vi "Main-top_feature.vi"() -> ()   [LabVIEW 2015]
uses:
  <vilib>/Utility/file.llb/Read Delimited Spreadsheet (string).vi
  <vilib>/Utility/file.llb/Write Delimited Spreadsheet (string).vi
  <vilib>/vision/NI_Vision_Development_Module.lvlib
  greenDet.dll
panel:
  out "element":string
  in  "Date Path":path=path "K:/Sort/TV/path - 副本.txt"
  in  "Image Main Path":path=path "K:/Sort/TV"
  in  "Save Base Path":path=path "K:/Sort/TV/1-Result"
  out "交集图":T1(plugin-control)
  out "交集像素个数":dbl
  in  "Pixel Measurements 2":T2[](array[typedef])=[35] items=["Center of Mass X", "Center of Mass Y", "First Pixel X", "First Pixel Y", "Bounding Rect Left", "Bounding Rect Top", "Bounding Rect Right", "Bounding Rect Bottom", "Max Feret Diameter Start X", "Max Feret Diameter Start Y", "Max Feret Diameter End X", "Max Feret Diameter End Y", "Max Horiz. Segment Length Left", "Max Horiz. Segment Length Right", "Max Horiz. Segment Length Row", "-", "Bounding Rect Width", "Bounding Rect Height", "Bounding Rect Diagonal", "Perimeter", "Convex Hull Perimeter", "Holes' Perimeter", "Max Feret Diameter", "Equivalent Ellipse Major Axis", "Equivalent Ellipse Minor Axis", "Equivalent Ellipse Minor Axis (Feret)", "Equivalent Rect Long Side", "Equivalent Rect Short Side", "Equivalent Rect Diagonal", "Equivalent Rect Short Side (Feret)", "Average Horiz. Segment Length", "Average Vert. Segment Length", "Hydraulic Radius", "Waddel Disk Diameter", "-", "Area", "Holes' Area", "Particle & Holes' Area", "Convex Hull Area", "Image Area", "-", "Number of Holes", "Number of Horiz. Segments", "Number of Vert. Segments", "-", "Orientation", "Max Feret Diameter Orientation", "-", "% Area/Image Area", "% Area/(Particle & Holes' Area)", "Ratio of Equivalent Ellipse Axes", "Ratio of Equivalent Rect Sides", "-", "Elongation Factor", "Compactness Factor", "Heywood Circularity Factor", "Type Factor", "-", "Sum X", "Sum Y", "Sum XX", "Sum XY", "Sum YY", "Sum XXX", "Sum XXY", "Sum XYY", "Sum YYY", "-", "Moment of Inertia XX", "Moment of Inertia XY", "Moment of Inertia YY", "Moment of Inertia XXX", "Moment of Inertia XXY", "Moment of Inertia XYY", "Moment of Inertia YYY", "Norm. Moment of Inertia XX", "Norm. Moment of Inertia XY", "Norm. Moment of Inertia YY", "Norm. Moment of Inertia XXX", "Norm. Moment of Inertia XXY", "Norm. Moment of Inertia XYY", "Norm. Moment of Inertia YYY", "Hu Moment 1", "Hu Moment 2", "Hu Moment 3", "Hu Moment 4", "Hu Moment 5", "Hu Moment 6", "Hu Moment 7"]
  in  "Pixel Measurements":T2[](array[typedef])=[35] items=["Center of Mass X", "Center of Mass Y", "First Pixel X", "First Pixel Y", "Bounding Rect Left", "Bounding Rect Top", "Bounding Rect Right", "Bounding Rect Bottom", "Max Feret Diameter Start X", "Max Feret Diameter Start Y", "Max Feret Diameter End X", "Max Feret Diameter End Y", "Max Horiz. Segment Length Left", "Max Horiz. Segment Length Right", "Max Horiz. Segment Length Row", "-", "Bounding Rect Width", "Bounding Rect Height", "Bounding Rect Diagonal", "Perimeter", "Convex Hull Perimeter", "Holes' Perimeter", "Max Feret Diameter", "Equivalent Ellipse Major Axis", "Equivalent Ellipse Minor Axis", "Equivalent Ellipse Minor Axis (Feret)", "Equivalent Rect Long Side", "Equivalent Rect Short Side", "Equivalent Rect Diagonal", "Equivalent Rect Short Side (Feret)", "Average Horiz. Segment Length", "Average Vert. Segment Length", "Hydraulic Radius", "Waddel Disk Diameter", "-", "Area", "Holes' Area", "Particle & Holes' Area", "Convex Hull Area", "Image Area", "-", "Number of Holes", "Number of Horiz. Segments", "Number of Vert. Segments", "-", "Orientation", "Max Feret Diameter Orientation", "-", "% Area/Image Area", "% Area/(Particle & Holes' Area)", "Ratio of Equivalent Ellipse Axes", "Ratio of Equivalent Rect Sides", "-", "Elongation Factor", "Compactness Factor", "Heywood Circularity Factor", "Type Factor", "-", "Sum X", "Sum Y", "Sum XX", "Sum XY", "Sum YY", "Sum XXX", "Sum XXY", "Sum XYY", "Sum YYY", "-", "Moment of Inertia XX", "Moment of Inertia XY", "Moment of Inertia YY", "Moment of Inertia XXX", "Moment of Inertia XXY", "Moment of Inertia XYY", "Moment of Inertia YYY", "Norm. Moment of Inertia XX", "Norm. Moment of Inertia XY", "Norm. Moment of Inertia YY", "Norm. Moment of Inertia XXX", "Norm. Moment of Inertia XXY", "Norm. Moment of Inertia XYY", "Norm. Moment of Inertia YYY", "Hu Moment 1", "Hu Moment 2", "Hu Moment 3", "Hu Moment 4", "Hu Moment 5", "Hu Moment 6", "Hu Moment 7"]
  out "黄色分量（油菜花）二值图":T1(plugin-control)
  out "黄色分量（油菜花）":T1(plugin-control)
  out "Original Image":T1(plugin-control)
  out "Current Path":path
  out "Current Number":string
  in  "ROI_whole":T3={"Top"=550, "im_height"=1000, "L_left"=650, "im_width"=1050}
  in  "Crop image ?":bool
  out "HistStat_whole":dbl[](array[numeric])
  out "AC (Area Convexity)":dbl
  out "P":dbl
  out "TPA (Total projective area)":dbl
  out "SFD":sgl
  out "BW (minimum circumscribed box width)":dbl
  out "BH":dbl
  out "R (Rectangularity)":dbl
  out "IFD":sgl
  out "Hull area":dbl
  out "HWR":dbl
  out "greenDet":dbl
  out "Crop Image":T1(plugin-control)
  out "Binary Image":T1(plugin-control)
  in  "EG threshold":sgl=0.2
  in  "ER threshold":sgl=0.5
  out "移除小区域后图像":T1(plugin-control)
  out "叶片分割后图像":T1(plugin-control)
  out "GPA (Green projective area)":dbl
  out "YPA (Yellow projective area)":dbl
  out "Image Path":path
  # "Digital evaluation software for oilseed rape phenotype-related traits (top-view) v1.0"
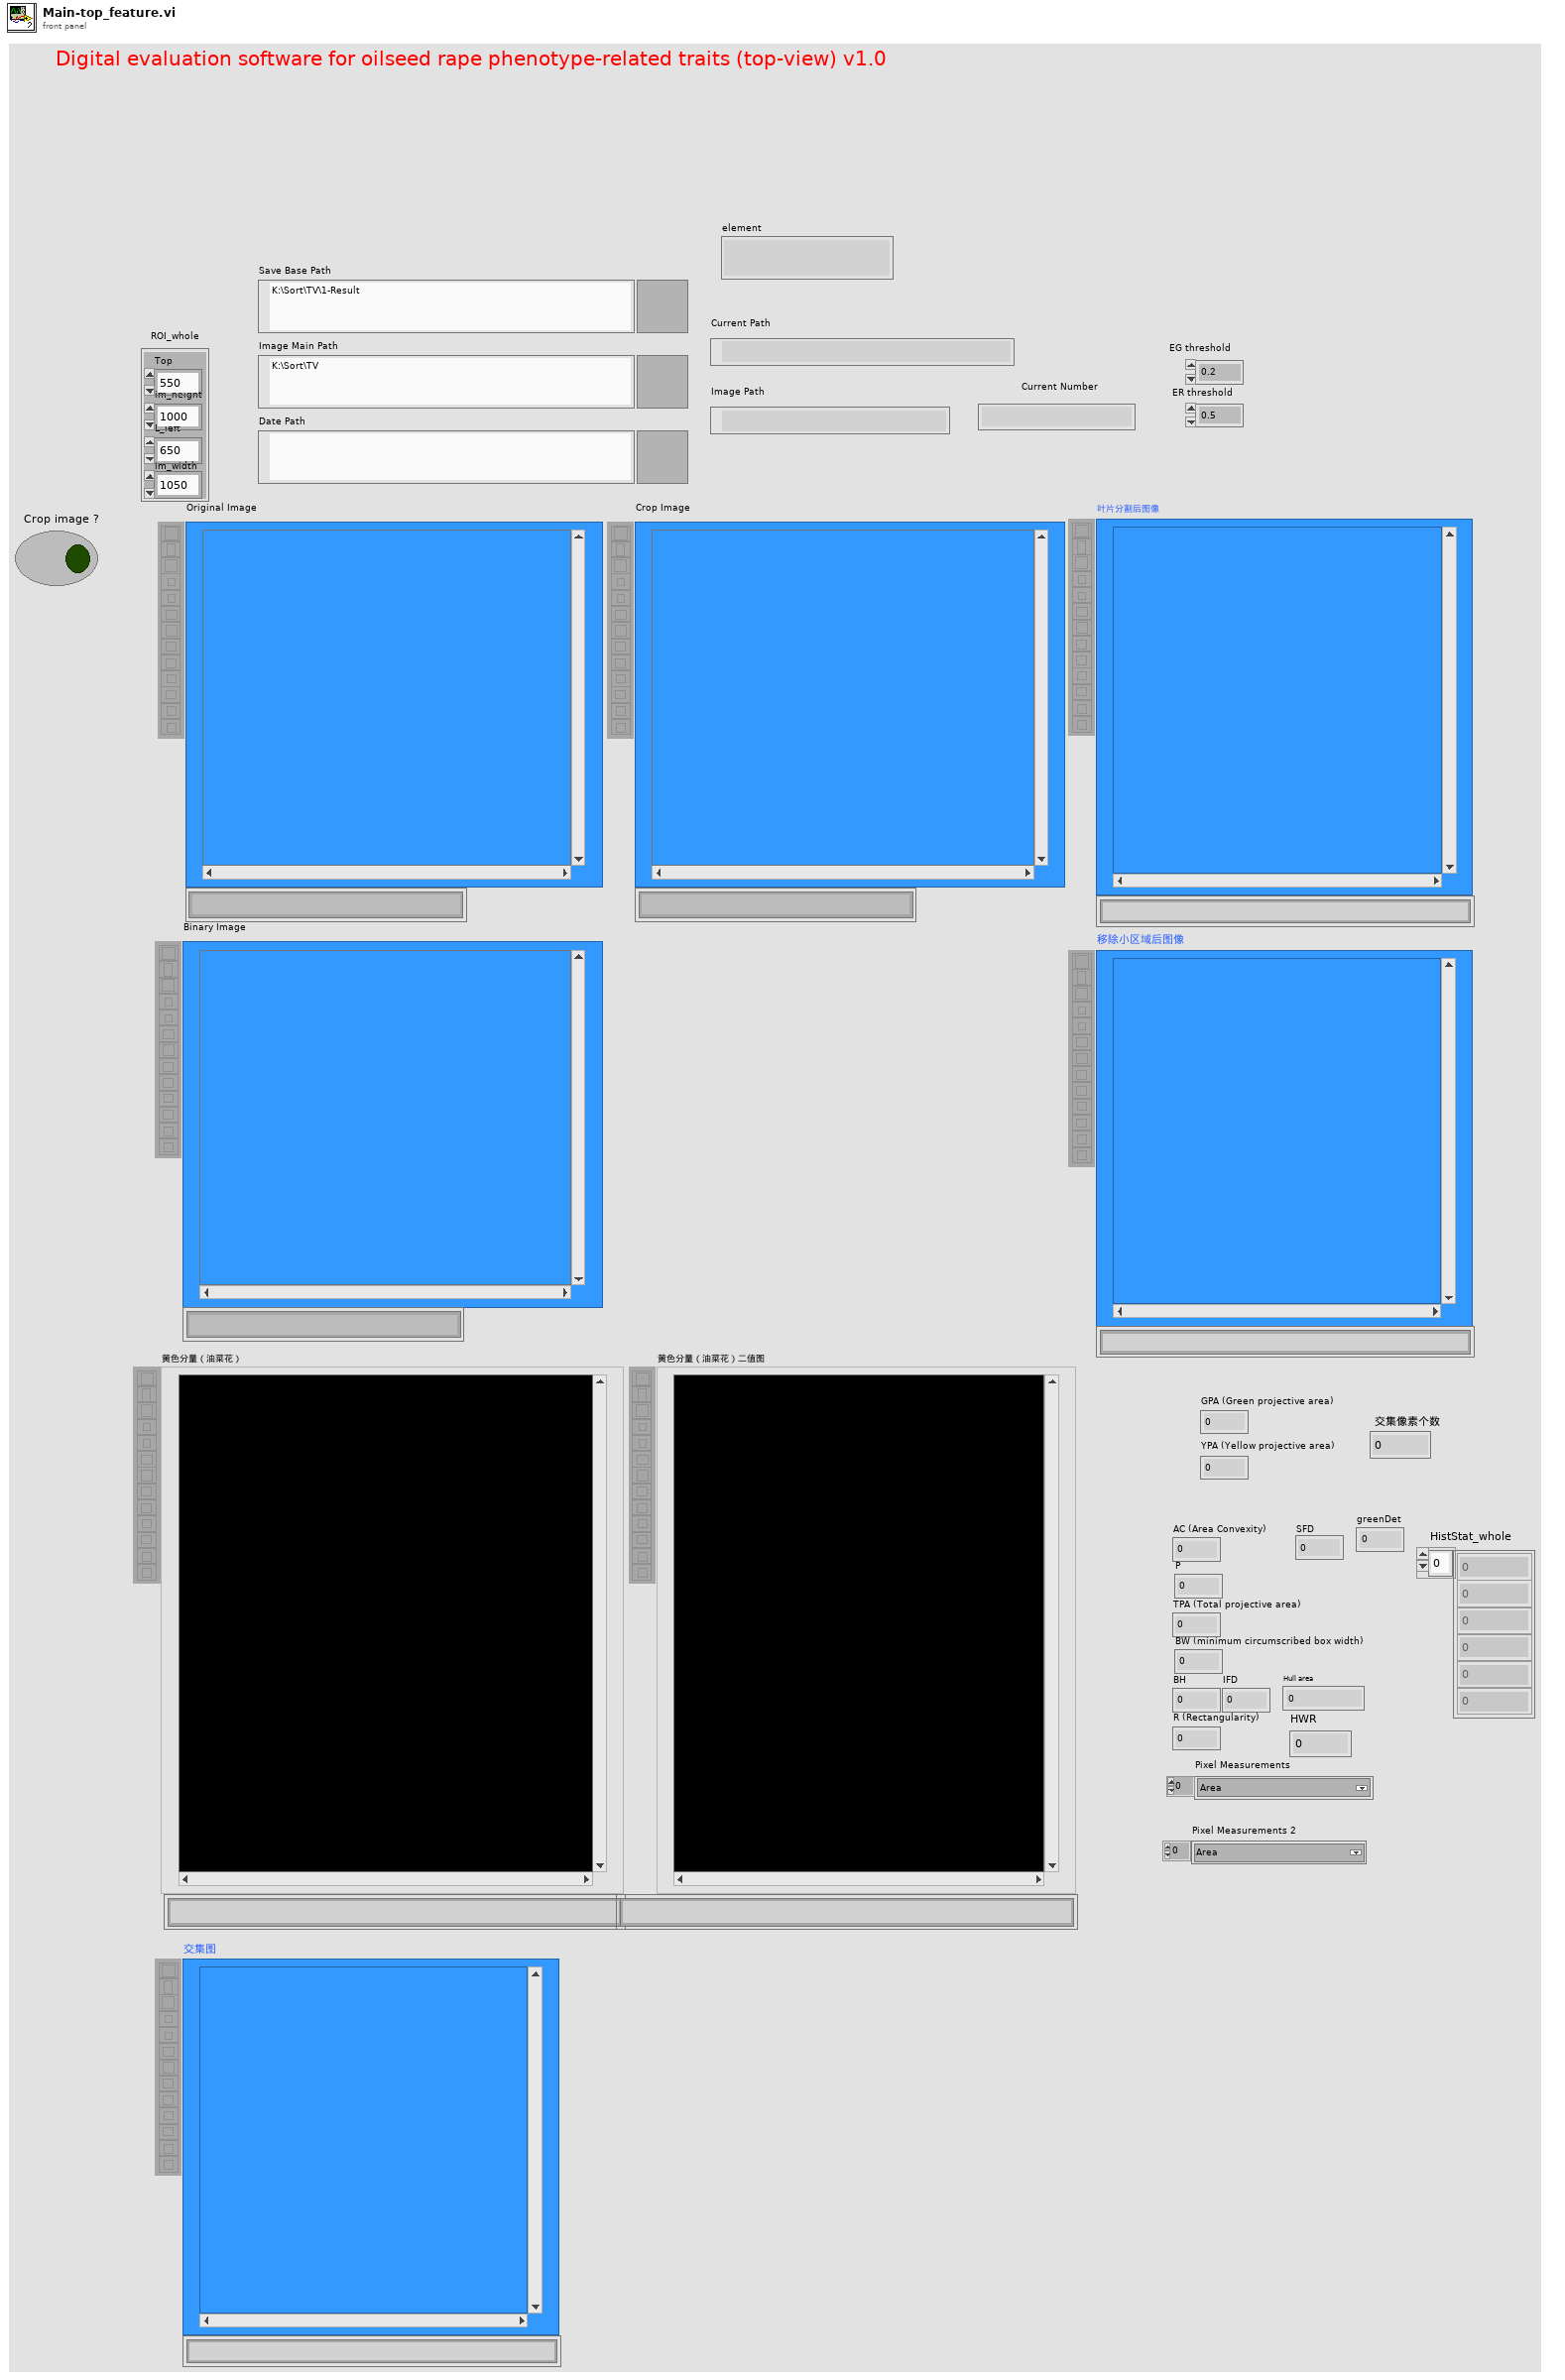
[diagram p1: front panel]
types:
  T1 = typedef "IMAQ Image.ctl" = refnum<image>
  T2 = typedef "Particle Parameters" = i32
  T3 = cluster{"Top":i32, "im_height":i32, "L_left":i32, "im_width":i32}
  T4 = enum32{"AutoM", "Close", "Dilate", "Erode", "Gradient", "Gradient out", "Gradient in", "Hit miss", "Open", "PClose", "POpen", "Thick", "Thin"}
  T5 = typedef "Image Type" = u32
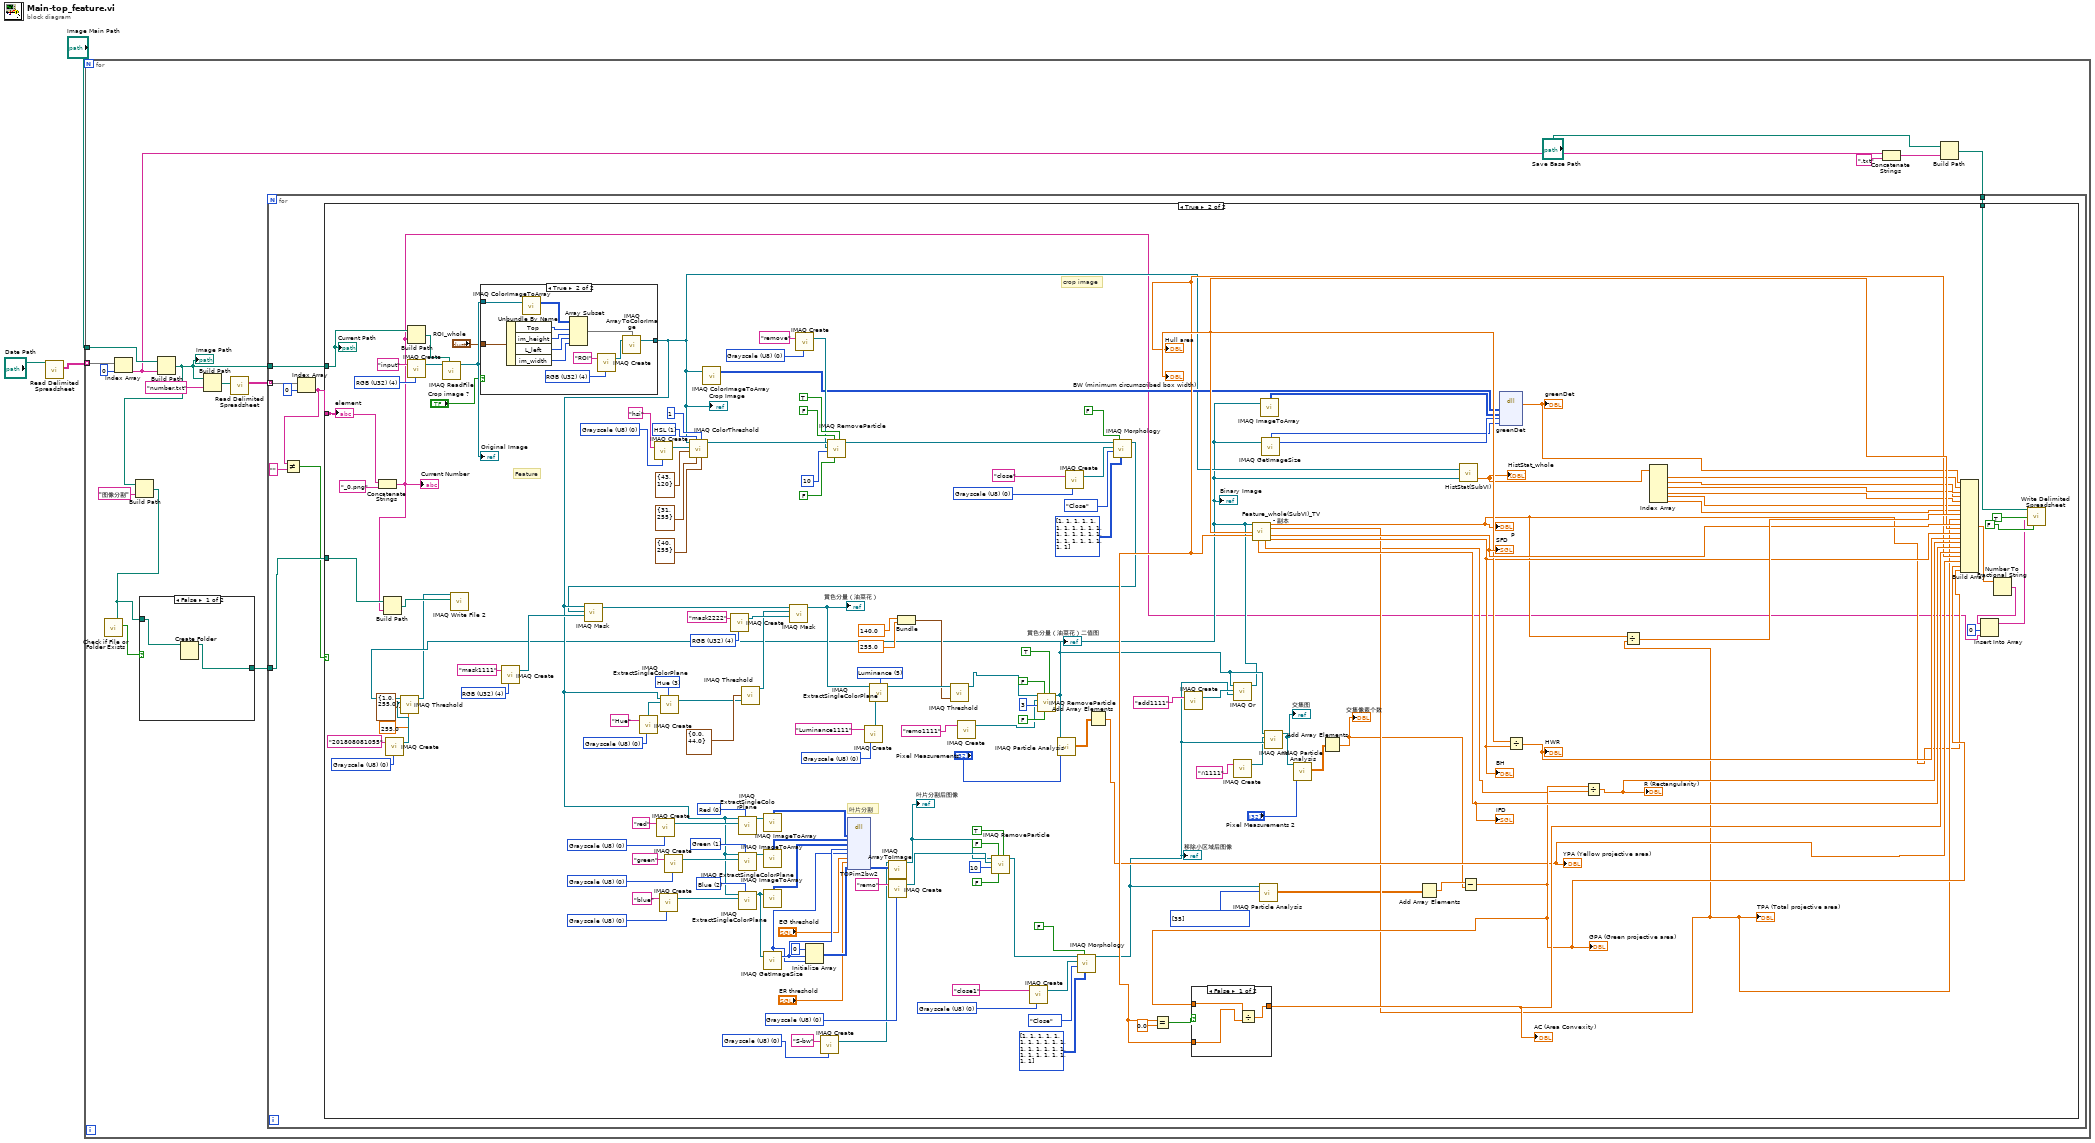
[diagram p0: block diagram]
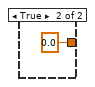
[diagram p4: hidden frame]
diagram:
  n1 = call-poly <vilib>:"Read Delimited Spreadsheet.vi"("file path (dialog if empty)"="Date Path") -> ("all rows"=w1:string[][])  [unwired: 9 in, 5 out]
  n2 = for {
    tunnel: "Image Main Path" -> [w19]
    tunnel: w1 -> [w17] mode=indexing
    n3 = Index Array(array=w17, index=0) -> (element=w4:string)
    n4 = Build Path(base path=w19, name or relative path=w4) -> (appended path=w13:path)
    "Image Path" <- w13
    n5 = Build Path(base path=w13, name or relative path="图像分割") -> (appended path=w10:path)
    n6 = call <vilib>:"Check if File or Folder Exists.vi"("path"=w10) -> ("file or folder exists?"=w11:bool)  [unwired: 8 in, 2 out]
    n7 = case shown="False" w11 {
      tunnel: [w20 w22] -> w9
      tunnel: w10 -> [w21 w22]
      frame False {
        n8 = Create Folder(path (use dialog)=w21) -> (created path=w20:path)  [unwired: 2 in, 2 out]
      }
      frame True {
      }
    }
    n9 = Build Path(base path=w13, name or relative path="number.txt") -> (appended path=w15:path)
    n10 = call-poly <vilib>:"Read Delimited Spreadsheet.vi"("file path (dialog if empty)"=w15) -> ("all rows"=w14:string[][])  [unwired: 9 in, 5 out]
    n11 = Concatenate Strings(w4, ".txt" ("string")) -> (w7:string)
    n12 = Build Path(base path="Save Base Path", name or relative path=w7) -> (appended path=w5:path)
    n13 = for {
      tunnel: w13 -> [w28]
      tunnel: w14 -> [w29] mode=indexing
      tunnel: w9 -> [w27]
      tunnel: w5 -> [w26]
      n14 = Index Array(array=w29, index=0) -> (element=w25:string)
      n15 = Not Equal?(x=w25, y="") -> (x != y?=w23:bool)
      n16 = case shown="True" w23 {
        tunnel: w28 -> [_ w198]
        tunnel: w27 -> [_ w176]
        tunnel: w26 -> [_ w175]
        tunnel: w25 -> [_ w33]
        frame False {
        }
        frame True {
          w43 = u32 0 items=["Grayscale (U8)", "Grayscale (I16)", "Grayscale (SGL)", "Complex (CSG)", "RGB (U32)", "HSL (U32)", "RGB (U64)"] ("Image Type")
          w73 = u32 0 items=["Grayscale (U8)", "Grayscale (I16)", "Grayscale (SGL)", "Complex (CSG)", "RGB (U32)", "HSL (U32)", "RGB (U64)"] ("Image Type")
          w76 = 5 items=["Red", "Green", "Blue", "Hue", "Saturation", "Luminance", "Value", "Intensity"] ("Color Plane")
          w80 = u32 0 items=["Grayscale (U8)", "Grayscale (I16)", "Grayscale (SGL)", "Complex (CSG)", "RGB (U32)", "HSL (U32)", "RGB (U64)"] ("Image Type")
          w83 = 3 items=["Red", "Green", "Blue", "Hue", "Saturation", "Luminance", "Value", "Intensity"] ("Color Plane")
          w86 = u32 4 items=["Grayscale (U8)", "Grayscale (I16)", "Grayscale (SGL)", "Complex (CSG)", "RGB (U32)", "HSL (U32)", "RGB (U64)"] ("Image Type")
          w89 = u32 4 items=["Grayscale (U8)", "Grayscale (I16)", "Grayscale (SGL)", "Complex (CSG)", "RGB (U32)", "HSL (U32)", "RGB (U64)"] ("Image Type")
          w98 = u32 0 items=["Grayscale (U8)", "Grayscale (I16)", "Grayscale (SGL)", "Complex (CSG)", "RGB (U32)", "HSL (U32)", "RGB (U64)"] ("Image Type")
          w102 = T2[] [35] items=["Center of Mass X", "Center of Mass Y", "First Pixel X", "First Pixel Y", "Bounding Rect Left", "Bounding Rect Top", "Bounding Rect Right", "Bounding Rect Bottom", "Max Feret Diameter Start X", "Max Feret Diameter Start Y", "Max Feret Diameter End X", "Max Feret Diameter End Y", "Max Horiz. Segment Length Left", "Max Horiz. Segment Length Right", "Max Horiz. Segment Length Row", "-", "Bounding Rect Width", "Bounding Rect Height", "Bounding Rect Diagonal", "Perimeter", "Convex Hull Perimeter", "Holes' Perimeter", "Max Feret Diameter", "Equivalent Ellipse Major Axis", "Equivalent Ellipse Minor Axis", "Equivalent Ellipse Minor Axis (Feret)", "Equivalent Rect Long Side", "Equivalent Rect Short Side", "Equivalent Rect Diagonal", "Equivalent Rect Short Side (Feret)", "Average Horiz. Segment Length", "Average Vert. Segment Length", "Hydraulic Radius", "Waddel Disk Diameter", "-", "Area", "Holes' Area", "Particle & Holes' Area", "Convex Hull Area", "Image Area", "-", "Number of Holes", "Number of Horiz. Segments", "Number of Vert. Segments", "-", "Orientation", "Max Feret Diameter Orientation", "-", "% Area/Image Area", "% Area/(Particle & Holes' Area)", "Ratio of Equivalent Ellipse Axes", "Ratio of Equivalent Rect Sides", "-", "Elongation Factor", "Compactness Factor", "Heywood Circularity Factor", "Type Factor", "-", "Sum X", "Sum Y", "Sum XX", "Sum XY", "Sum YY", "Sum XXX", "Sum XXY", "Sum XYY", "Sum YYY", "-", "Moment of Inertia XX", "Moment of Inertia XY", "Moment of Inertia YY", "Moment of Inertia XXX", "Moment of Inertia XXY", "Moment of Inertia XYY", "Moment of Inertia YYY", "Norm. Moment of Inertia XX", "Norm. Moment of Inertia XY", "Norm. Moment of Inertia YY", "Norm. Moment of Inertia XXX", "Norm. Moment of Inertia XXY", "Norm. Moment of Inertia XYY", "Norm. Moment of Inertia YYY", "Hu Moment 1", "Hu Moment 2", "Hu Moment 3", "Hu Moment 4", "Hu Moment 5", "Hu Moment 6", "Hu Moment 7"] ("Pixel Measurements")
          w136 = T5 0 items=["Grayscale (U8)", "Grayscale (I16)", "Grayscale (SGL)", "Complex (CSG)", "RGB (U32)", "HSL (U32)", "RGB (U64)", "Grayscale (U16)"] ("Image Type")
          w129 = T5 0 items=["Grayscale (U8)", "Grayscale (I16)", "Grayscale (SGL)", "Complex (CSG)", "RGB (U32)", "HSL (U32)", "RGB (U64)", "Grayscale (U16)"] ("Image Type")
          w115 = 2 items=["Red", "Green", "Blue", "Hue", "Saturation", "Luminance", "Value", "Intensity"] ("Color Plane")
          w114 = 0 items=["Red", "Green", "Blue", "Hue", "Saturation", "Luminance", "Value", "Intensity"] ("Color Plane")
          w111 = T5 0 items=["Grayscale (U8)", "Grayscale (I16)", "Grayscale (SGL)", "Complex (CSG)", "RGB (U32)", "HSL (U32)", "RGB (U64)", "Grayscale (U16)"] ("Image Type")
          w109 = 1 items=["Red", "Green", "Blue", "Hue", "Saturation", "Luminance", "Value", "Intensity"] ("Color Plane")
          w106 = T5 0 items=["Grayscale (U8)", "Grayscale (I16)", "Grayscale (SGL)", "Complex (CSG)", "RGB (U32)", "HSL (U32)", "RGB (U64)", "Grayscale (U16)"] ("Image Type")
          w110 = T5 0 items=["Grayscale (U8)", "Grayscale (I16)", "Grayscale (SGL)", "Complex (CSG)", "RGB (U32)", "HSL (U32)", "RGB (U64)", "Grayscale (U16)"] ("Image Type")
          w140 = u32 0 items=["Grayscale (U8)", "Grayscale (I16)", "Grayscale (SGL)", "Complex (CSG)", "RGB (U32)", "HSL (U32)", "RGB (U64)"] ("Image Type")
          w152 = u32 0 items=["Grayscale (U8)", "Grayscale (I16)", "Grayscale (SGL)", "Complex (CSG)", "RGB (U32)", "HSL (U32)", "RGB (U64)"] ("Image Type")
          w155 = u32 0 items=["Grayscale (U8)", "Grayscale (I16)", "Grayscale (SGL)", "Complex (CSG)", "RGB (U32)", "HSL (U32)", "RGB (U64)"] ("Image Type")
          w157 = u16 1 items=["RGB", "HSL", "HSV", "HSI"] ("Color Mode")
          w172 = T5 4 items=["Grayscale (U8)", "Grayscale (I16)", "Grayscale (SGL)", "Complex (CSG)", "RGB (U32)", "HSL (U32)", "RGB (U64)", "Grayscale (U16)"] ("Image Type")
          # "叶片分割"
          # "crop image"
          # "Feature"
          n17 = Concatenate Strings(w33, "_0.png" ("string")) -> (w31:string)
          "Current Number" <- w31
          n18 = Build Path(base path=w176, name or relative path=w31) -> (appended path=w45:path)
          n19 = call "IMAQ Create"("Image Name"="201808081055", "Image Type"=w43) -> ("New Image"=w41:T1)  [unwired: 2 in, 2 out]
          n20 = Build Path(base path=w198, name or relative path=w31) -> (appended path=w171:path)
          n21 = call "IMAQ Create"("Image Name"="input", "Image Type"=w172) -> ("New Image"=w173:T1)  [unwired: 2 in, 2 out]
          n22 = call "IMAQ ReadFile"("File Path"=w171, "Image"=w173) -> ("Image Out"=w169:T1)  [unwired: 3 in, 6 out]
          "Original Image" <- w169
          n23 = case shown="True" "Crop image ?" {
            tunnel: w169 -> [w203 w210]
            tunnel: "ROI_whole" -> [_ w205]
            tunnel: [w203 w204] -> w58
            frame False {
            }
            frame True {
              w208 = u32 4 items=["Grayscale (U8)", "Grayscale (I16)", "Grayscale (SGL)", "Complex (CSG)", "RGB (U32)", "HSL (U32)", "RGB (U64)"] ("Image Type")
              n24 = Unbundle By Name(w205) -> ("Top"=w212:i32, "im_height"=w213:i32, "L_left"=w214:i32, "im_width"=w215:i32)
              n25 = call "IMAQ ColorImageToArray"("Image"=w210) -> ("Image Pixels (U32)"=w211:u32[][])  [unwired: 2 in, 3 out]
              n26 = Array Subset(array=w211, index (row)=w212, length (row)=w213, index (col)=w214, length (col)=w215) -> (w206:u32[][])
              n27 = call "IMAQ Create"("Image Name"="ROI", "Image Type"=w208) -> ("New Image"=w207:T1)  [unwired: 2 in, 2 out]
              n28 = call "IMAQ ArrayToColorImage"("Image Pixels (U32)"=w206, "Image"=w207) -> ("Image Out"=w204:T1)  [unwired: 2 in, 2 out]
            }
          }
          "Crop Image" <- w58
          n29 = call "IMAQ Create"("Image Name"="mask1111", "Image Type"=w89) -> ("New Image"=w88:T1)  [unwired: 2 in, 2 out]
          n30 = call "IMAQ Create"("Image Name"="Hue", "Image Type"=w80) -> ("New Image"=w79:T1)  [unwired: 2 in, 2 out]
          n31 = call "IMAQ Create"("Image Name"="hsi", "Image Type"=w155) -> ("New Image"=w154:T1)  [unwired: 2 in, 2 out]
          n32 = call "IMAQ Create"("Image Name"="red", "Image Type"=w110) -> ("New Image"=w105:T1)  [unwired: 2 in, 2 out]
          n33 = call "IMAQ Create"("Image Name"="blue", "Image Type"=w106) -> ("New Image"=w108:T1)  [unwired: 2 in, 2 out]
          n34 = call "IMAQ ExtractSingleColorPlane"("Color Plane"=w83, "Image Dst"=w79, "Image Src"=w58) -> ("Image Dst Out"=w81:T1)  [unwired: 1 in, 7 out]
          n35 = call "IMAQ Create"("Image Name"="green", "Image Type"=w111) -> ("New Image"=w113:T1)  [unwired: 2 in, 2 out]
          n36 = call "IMAQ ColorThreshold"("Blue or Luma or Val or Inten Range"=cluster{"Lower value":i32, "Upper value":i32} {"Lower value"=40, "Upper value"=255}, "Replace Value"=1, "Green or Sat Range"=cluster{"Lower value":i32, "Upper value":i32} {"Lower value"=31, "Upper value"=255}, "Color Mode"=w157, "Red or Hue Range"=cluster{"Lower value":i32, "Upper value":i32} {"Lower value"=43, "Upper value"=120}, "Image Dst"=w154, "Image Src"=w58) -> ("Image Dst Out"=w158:T1)  [unwired: 1 in, 3 out]
          n37 = call "IMAQ ColorImageToArray"("Image"=w58) -> ("Image Pixels (U32)"=w150:u32[][])  [unwired: 2 in, 3 out]
          n38 = call "IMAQ Create"("Image Name"="mask2222", "Image Type"=w86) -> ("New Image"=w85:T1)  [unwired: 2 in, 2 out]
          n39 = call "IMAQ ExtractSingleColorPlane"("Color Plane"=w114, "Image Dst"=w105, "Image Src"=w58) -> ("Image Dst Out"=w117:T1)  [unwired: 1 in, 7 out]
          n40 = call "IMAQ ExtractSingleColorPlane"("Color Plane"=w109, "Image Dst"=w113, "Image Src"=w58) -> ("Image Dst Out"=w116:T1)  [unwired: 1 in, 7 out]
          n41 = call "IMAQ ExtractSingleColorPlane"("Color Plane"=w115, "Image Dst"=w108, "Image Src"=w58) -> ("Image Dst Out"=w121:T1)  [unwired: 1 in, 7 out]
          n42 = call "IMAQ Threshold"("Range"=cluster{"Lower value":sgl, "Upper value":sgl} {"Lower value"=0.0, "Upper value"=44.0}, "Image Src"=w81) -> ("Image Dst Out"=w59:T1)  [unwired: 4 in, 5 out]
          n43 = call "IMAQ ImageToArray"("Image"=w117) -> ("Image Pixels (U8)"=w119:u8[][])  [unwired: 2 in, 5 out]
          n44 = call "IMAQ ImageToArray"("Image"=w116) -> ("Image Pixels (U8)"=w118:u8[][])  [unwired: 2 in, 5 out]
          n45 = call "IMAQ ImageToArray"("Image"=w121) -> ("Image Pixels (U8)"=w120:u8[][])  [unwired: 2 in, 5 out]
          n46 = call "IMAQ GetImageSize"("Image"=w121) -> ("Y Resolution"=w126:i32, "X Resolution"=w125:i32)  [unwired: 1 in, 3 out]
          n47 = call "IMAQ Create"("Image Name"="remove", "Image Type"=w152) -> ("New Image"=w151:T1)  [unwired: 2 in, 2 out]
          n48 = Initialize Array(u8 0 ("element"), w126, w125) -> (w127:u8[][])
          n49 = call "IMAQ Create"("Image Name"="S-bw", "Image Type"=w129) -> ("New Image"=w130:T1)  [unwired: 2 in, 2 out]
          n50 = call "IMAQ RemoveParticle"("Connectivity 4/8 (8)"=TRUE, "Low Pass/High Pass (Low)"=FALSE, "Square/Hexa (Square)"=FALSE, "Number of Erosion"=10, "Image Dst"=w151, "Image Src"=w158) -> ("Image Dst Out"=w142:T1)  [unwired: 1 in, 4 out]
          n51 = dll-call lib="PTH2¢abs Dfhä¼ è¾E\tRPAE Workæç®éè¯»æ²¹è æç«  ææµ·æ¶ææµ·æ¶oilseedRape measurement proceduresæ²¹èé¡¶è§d..." fn="TOPim2bw2"("R"=w119, "G"=w118, "B"=w120, "row"=w126, "col"=w125, "EGthreshold"="EG threshold", "ERthreshold"="ER threshold", "bw"=w127) -> ("bw"=w131:u8[][])  [unwired: 10 in, 3 out]
          n52 = call "IMAQ Create"("Image Name"="Luminance1111", "Image Type"=w73) -> ("New Image"=w75:T1)  [unwired: 2 in, 2 out]
          n53 = call "IMAQ ArrayToImage"("Image Pixels (U8)"=w131, "Image"=w130) -> ("Image Out"=w95:T1)  [unwired: 4 in, 5 out]
          "叶片分割后图像" <- w95
          n54 = call "IMAQ Create"("Image Name"="remo", "Image Type"=w136) -> ("New Image"=w138:T1)  [unwired: 2 in, 2 out]
          n55 = Bundle("Lower value"=sgl 140.0, "Upper value"=sgl 255.0) -> (w69:cluster{"Lower value":sgl, "Upper value":sgl})  [unwired: 1 in]
          n56 = call "IMAQ Create"("Image Name"="remo1111") -> ("New Image"=w62:T1)  [unwired: 3 in, 2 out]
          n57 = call "IMAQ RemoveParticle"("Connectivity 4/8 (8)"=TRUE, "Low Pass/High Pass (Low)"=FALSE, "Square/Hexa (Square)"=FALSE, "Number of Erosion"=10, "Image Dst"=w138, "Image Src"=w95) -> ("Image Dst Out"=w94:T1)  [unwired: 1 in, 4 out]
          n58 = call "IMAQ Create"("Image Name"="close1", "Image Type"=w98) -> ("New Image"=w97:T1)  [unwired: 2 in, 2 out]
          n59 = call "IMAQ Create"("Image Name"="close", "Image Type"=w140) -> ("New Image"=w139:T1)  [unwired: 2 in, 2 out]
          n60 = call "IMAQ Morphology"("Structuring Element"=i32[][] [[1, 1, 1, 1, 1], [1, 1, 1, 1, 1], [1, 1, 1, 1, 1], [1, 1, 1, 1, 1], [1, 1, 1, 1, 1]], "Square/Hexa (Square)"=FALSE, "Operation"=T4."Close", "Image Dst"=w97, "Image Src"=w94) -> ("Image Dst Out"=w53:T1)  [unwired: 2 in, 4 out]
          "移除小区域后图像" <- w53
          n61 = call "IMAQ Morphology"("Structuring Element"=i32[][] [[1, 1, 1, 1, 1], [1, 1, 1, 1, 1], [1, 1, 1, 1, 1], [1, 1, 1, 1, 1], [1, 1, 1, 1, 1]], "Square/Hexa (Square)"=FALSE, "Operation"=T4."Close", "Image Dst"=w139, "Image Src"=w142) -> ("Image Dst Out"=w56:T1)  [unwired: 2 in, 4 out]
          n62 = call "IMAQ Mask"("Image Dst"=w88, "Image Mask"=w56, "Image Src"=w58) -> ("Image Dst Out"=w84:T1)  [unwired: 1 in, 2 out]
          n63 = call "IMAQ Mask"("Image Dst"=w85, "Image Mask"=w59, "Image Src"=w84) -> ("Image Dst Out"=w74:T1)  [unwired: 1 in, 2 out]
          "黄色分量（油菜花）" <- w74
          n64 = call "IMAQ ExtractSingleColorPlane"("Color Plane"=w76, "Image Dst"=w75, "Image Src"=w74) -> ("Image Dst Out"=w77:T1)  [unwired: 1 in, 7 out]
          n65 = call "IMAQ Threshold"("Range"=w69, "Image Src"=w77) -> ("Image Dst Out"=w61:T1)  [unwired: 4 in, 5 out]
          n66 = call "IMAQ RemoveParticle"("Connectivity 4/8 (8)"=TRUE, "Low Pass/High Pass (Low)"=FALSE, "Square/Hexa (Square)"=FALSE, "Number of Erosion"=3, "Image Dst"=w62, "Image Src"=w61) -> ("Image Dst Out"=w54:T1)  [unwired: 1 in, 4 out]
          "黄色分量（油菜花）二值图" <- w54
          n67 = call "IMAQ Particle Analysis"("Pixel Measurements"="Pixel Measurements", "Image"=w54) -> ("Particle Measurements (Pixels)"=w68:dbl[][])  [unwired: 3 in, 6 out]
          n68 = Add Array Elements(numeric array=w68) -> (sum=w179:dbl)
          "YPA (Yellow projective area)" <- w179
          n69 = call "IMAQ Create"("Image Name"="add1111") -> ("New Image"=w55:T1)  [unwired: 3 in, 2 out]
          n70 = call "IMAQ Or"("Image Src B"=w53, "Image Dst"=w55, "Image Src A"=w54) -> ("Image Dst Out"=w44:T1)  [unwired: 7 in, 1 out]
          "Binary Image" <- w44
          n71 = call "IMAQ Threshold"("Replace Value"=sgl 255.0, "Range"=cluster{"Lower value":sgl, "Upper value":sgl} {"Lower value"=1.0, "Upper value"=255.0}, "Image Dst"=w41, "Image Src"=w44) -> ("Image Dst Out"=w38:T1)  [unwired: 6 in, 1 out]
          n72 = call-poly "IMAQ Write File 2"("File Path"=w45, "Image"=w38) -> ()  [unwired: 8 in, 2 out]
          n73 = call "IMAQ Create"("Image Name"="∩1111") -> ("New Image"=w51:T1)  [unwired: 3 in, 2 out]
          n74 = call "Feature_whole(SubVI)_TV - 副本.vi"("Binary Image"=w44) -> ("P"=w177:dbl, "SA"=w178:dbl, "SFD"=w196:sgl, "Hull area"=w189:dbl, "SW"=w195:dbl, "IFD"=w191:sgl, "最小外接矩面积"=w93:dbl, "SH"=w194:dbl)  [unwired: 6 in, 1 out]
          "P" <- w177
          "TPA (Total projective area)" <- w178
          "SFD" <- w196
          "BW (minimum circumscribed box width)" <- w195
          "BH" <- w194
          "IFD" <- w191
          "Hull area" <- w189
          n75 = Equal?(x=w189, y=0.0) -> (x = y?=w92:bool)
          n76 = call "IMAQ Particle Analysis"("Pixel Measurements"=w102, "Image"=w53) -> ("Particle Measurements (Pixels)"=w103:dbl[][])  [unwired: 3 in, 6 out]
          n77 = call "IMAQ ImageToArray"("Image"=w44) -> ("Image Pixels (U8)"=w149:u8[][])  [unwired: 2 in, 5 out]
          n78 = call "IMAQ GetImageSize"("Image"=w44) -> ("Y Resolution"=w148:i32, "X Resolution"=w147:i32)  [unwired: 1 in, 3 out]
          n79 = call "IMAQ And"("Image Src B"=w53, "Image Dst"=w51, "Image Src A"=w54) -> ("Image Dst Out"=w47:T1)  [unwired: 7 in, 1 out]
          "交集图" <- w47
          n80 = call "IMAQ Particle Analysis"("Pixel Measurements"="Pixel Measurements 2", "Image"=w47) -> ("Particle Measurements (Pixels)"=w50:dbl[][])  [unwired: 3 in, 6 out]
          n81 = Add Array Elements(numeric array=w50) -> (sum=w46:dbl)
          "交集像素个数" <- w46
          n82 = Add Array Elements(numeric array=w103) -> (sum=w48:dbl)
          n83 = call "HistStat(SubVI).vi"("Binary Image"=w44, "Original Image"=w58) -> ("HistStat"=w146:dbl[])  [unwired: 1 out]
          "HistStat_whole" <- w146
          n84 = Subtract(x=w48, y=w46) -> (x-y=w180:dbl)
          "GPA (Green projective area)" <- w180
          n85 = case shown="False" w92 {
            tunnel: w180 -> [w201 _]
            tunnel: w189 -> [w200 _]
            tunnel: [w199 0.0] -> w190
            frame False {
              n86 = Divide(x=w201, y=w200) -> (x/y=w199:dbl)
            }
            frame True {
            }
          }
          "AC (Area Convexity)" <- w190
          n87 = dll-call lib="PTH2abs Dfhä¼ è¾E\tRPAE Workæç®éè¯»æ²¹è æç«  ææµ·æ¶ææµ·æ¶oilseedRape measurement proceduresæ²¹èé¡¶è§top_featuresgreenDet.dll" fn="greenDet"("oriArray"=w150, "binArray"=w149, "imageRows"=w148, "imageCols"=w147) -> ("greenDet"=w188:dbl)  [unwired: 7 in, 2 out]
          "greenDet" <- w188
          n88 = Divide(x=w195, y=w194) -> (x/y=w193:dbl)
          "HWR" <- w193
          n89 = Divide(x=w180, y=w93) -> (x/y=w192:dbl)
          "R (Rectangularity)" <- w192
          n90 = Divide(x=w177, y=w178) -> (x/y=w197:dbl)
          n91 = Index Array(array=w146) -> (element #1=w187:dbl, element #2=w186:dbl, element #3=w185:dbl, element #4=w184:dbl, element #5=w183:dbl, element #6=w182:dbl)  [unwired: 6 in]
          n92 = Build Array(w188, w187, w186, w185, w184, w183, w182, w197, w178, w196, w195, w194, w193, w192, w191, w190, w189, w179, w180, w177) -> (w36:dbl[])
          n93 = Number To Fractional String(number=w36) -> (F-format string=w35:string[])  [unwired: 3 in]
          n94 = Insert Into Array(array=w35, index=0, new element=w31) -> (w32:string[])
          n95 = call-poly <vilib>:"Write Delimited Spreadsheet.vi"("file path (dialog if empty)"=w175, "1D data"=w32, "append to file? (F)"=TRUE, "transpose? (F)"=FALSE ("append to file? (new file:F)")) -> ()  [unwired: 10 in, 2 out]
          "Current Path" <- w198
          "element" <- w33
        }
      }
    }
  }
